vi "Parse Instructions.vi"(8 "error in (no error)":errorcluster, 11 "Instructions XML":string="<?xml version=\"1.0\" encoding=\"UTF-8\"?><ns2:instructions xmlns:ns2=\"http://jazz.net/xmlns/alm/qm/v0.1/\" xmlns:ns1=\"http://schema.ibm.com/vega/2008/\" xmlns:ns3=\"http://purl.org/dc/elements/1.1/\" xmlns:ns4=\"http://jazz.net/xmlns/prod/jazz/process/0.6/\" xmlns:ns5=\"http://jazz.net/xmlns/alm/v0.1/\" xmlns:ns6=\"http://www.w3.org/1999/02/22-rdf-syntax-ns#\" xmlns:ns7=\"http://purl.org/dc/terms/\" xmlns:ns8=\"http://jazz.net/xmlns/alm/qm/v0.1/tsl/v0.1/\" xmlns:ns9=\"http://jazz.net/xmlns/alm/qm/v0.1/testscript/v0.1/\" xmlns:ns10=\"http://jazz.net/xmlns/alm/qm/qmadapter/task/v0.1\" xmlns:ns11=\"http://jazz.net/xmlns/alm/qm/qmadapter/v0.1\" xmlns:ns12=\"http://jazz.net/xmlns/alm/qm/v0.1/executionworkitem/v0.1\" xmlns:ns13=\"http://jazz.net/xmlns/alm/qm/v0.1/executionresult/v0.1\" xmlns:ns14=\"http://jazz.net/xmlns/alm/qm/v0.1/catalog/v0.1\" xmlns:ns16=\"http://jazz.net/xmlns/alm/qm/styleinfo/v0.1/\" xmlns:ns17=\"http://www.w3.org/1999/XSL/Transform\"><ns11:workavailable>false</ns11:workavailable></ns2:instructions>") -> (0 "error out":errorcluster, 1 "Instructions":T1[](array[typedef]), 2 "Work available":bool)   [LabVIEW 2012]
uses:
  Instruction Info.ctl
  <vilib>/xml/Load XML String.vi
  <vilib>/xml/Close Reference(Node).vi
  <vilib>/xml/Close Reference(NdList).vi
  <vilib>/xml/NI_XML.lvlib
  <resource>/objmgr/DOMUserDefRef.rc
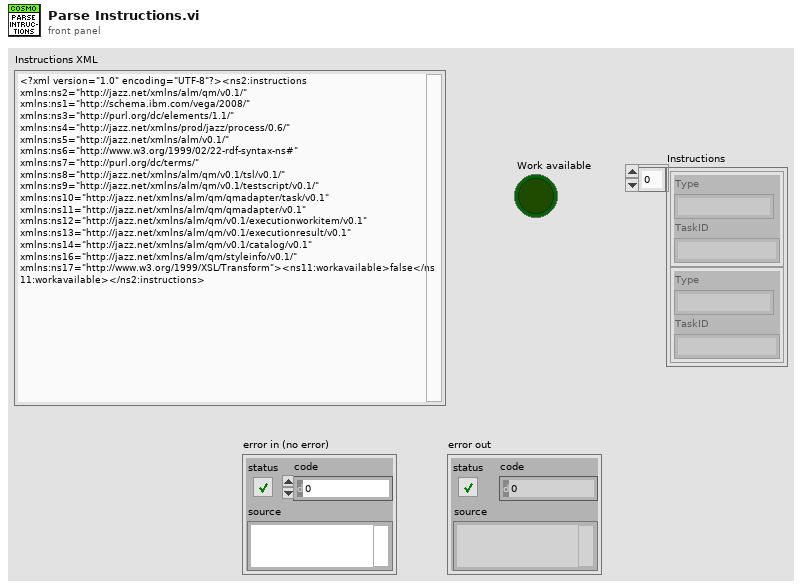
[diagram p1: front panel]
types:
  T1 = typedef "Instruction Info.ctl" = cluster{"Type":string, "TaskID":string}
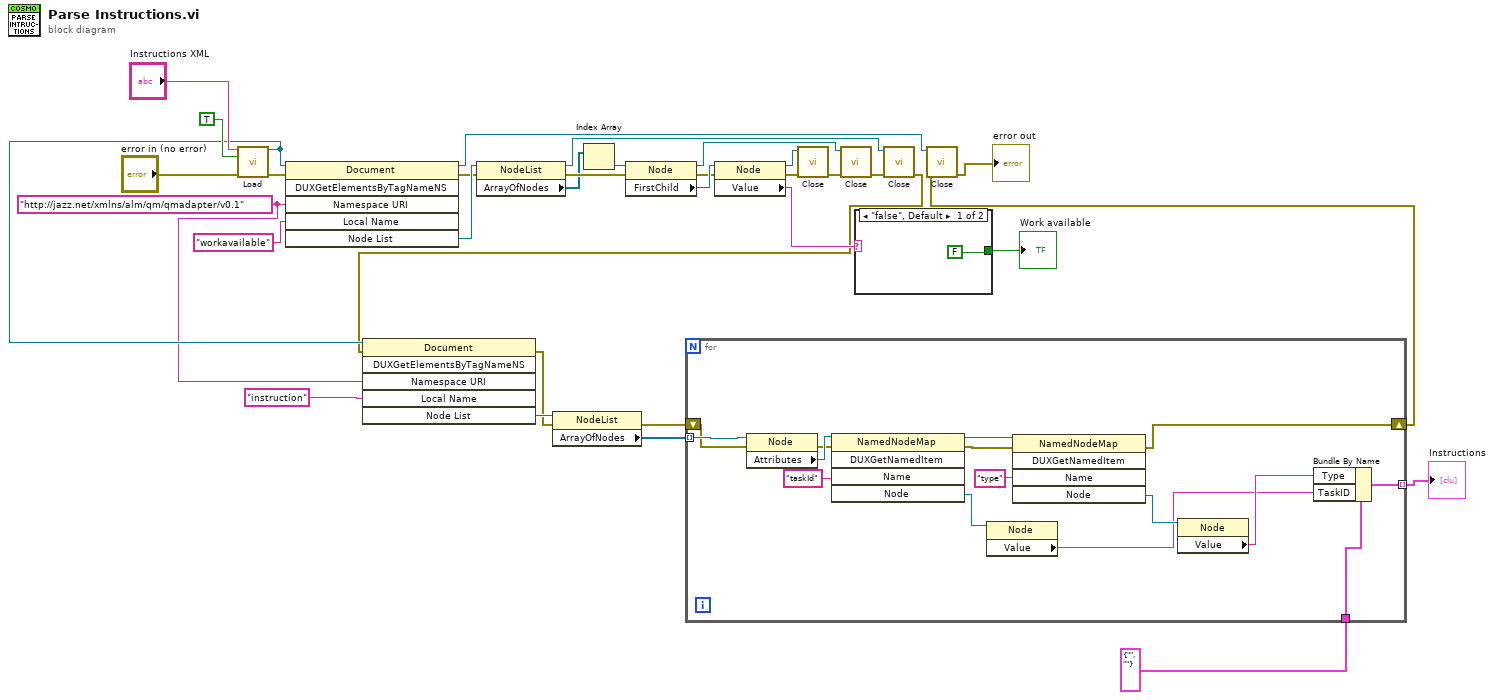
[diagram p0: block diagram]
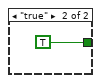
[diagram p2: hidden frame]
diagram:
  w11 = "http://jazz.net/xmlns/alm/qm/qmadapter/v0.1" ("Namespace URI")
  n1 = call-poly <vilib>:"Load.vi"("XML string"="Instructions XML", "process namespaces (False)"=TRUE, "error in (no error)"="error in (no error)") -> ("DOM document out"=w12:refnum<k20>, "error out"=w28:errorcluster)  [unwired: 10 in, 1 out]
  n2 = invoke class="Document" method="DUXGetElementsByTagNameNS"(reference=w12, error in=w28, "Namespace URI"=w11, "Local Name"="workavailable") -> (reference out=w21:refnum<k20>, error out=w29:errorcluster, "Node List"=w30:refnum<k20>)  [unwired: 2 in, 3 out]
  n3 = property class="NodeList"(reference=w30, error in=w29) -> (reference out=w27:refnum<k20>, error out=w24:errorcluster, "ArrayOfNodes"=w13:refnum<k20>[])
  n4 = Index Array(array=w13) -> (element=w25:refnum<k20>)  [unwired: 1 in]
  n5 = property class="Node"(reference=w25, error in=w24) -> (reference out=w22:refnum<k20>, error out=w19:errorcluster, "FirstChild"=w20:refnum<k20>)
  n6 = property class="Node"(reference=w20, error in=w19) -> (reference out=w18:refnum<k20>, error out=w17:errorcluster, "Value"=w15:string)
  n7 = call-poly <vilib>:"Close.vi"("error in (no error)"=w17, "node"=w18) -> ("error out"=w16:errorcluster)  [unwired: 7 in]
  n8 = call-poly <vilib>:"Close.vi"("error in (no error)"=w16, "node"=w22) -> ("error out"=w26:errorcluster)  [unwired: 7 in]
  n9 = case shown="\"false\", Default" w15 {
    tunnel: [FALSE TRUE] -> w14
    frame "false", Default {
    }
    frame "true" {
    }
  }
  "Work available" <- w14
  n10 = call-poly <vilib>:"Close.vi"("error in (no error)"=w26, "node list"=w27) -> ("error out"=w5:errorcluster)  [unwired: 7 in]
  n11 = invoke class="Document" method="DUXGetElementsByTagNameNS"(reference=w12, error in=w5, "Namespace URI"=w11, "Local Name"="instruction") -> (error out=w4:errorcluster, "Node List"=w9:refnum<k20>)  [unwired: 2 in, 4 out]
  n12 = property class="NodeList"(reference=w9, error in=w4) -> (error out=w3:errorcluster, "ArrayOfNodes"=w8:refnum<k20>[])  [unwired: 1 out]
  n13 = for {
    tunnel: w8 -> [w43] mode=indexing
    tunnel: T1 {"Type"="", "TaskID"=""} ("Intruction") -> [w42]
    tunnel: [w39] -> w6 mode=indexing
    shift-right: [w36] -> w2
    shift-left: w3 -> [w38]
    n14 = property class="Node"(reference=w43, error in=w38) -> (error out=w37:errorcluster, "Attributes"=w50:refnum<k20>)  [unwired: 1 out]
    n15 = invoke class="NamedNodeMap" method="DUXGetNamedItem"(reference=w50, error in=w37, "Name"="taskId") -> (reference out=w48:refnum<k20>, error out=w47:errorcluster, "Node"=w45:refnum<k20>)  [unwired: 2 in, 2 out]
    n16 = property class="Node"(reference=w45) -> ("Value"=w40:string)  [unwired: 1 in, 2 out]
    n17 = invoke class="NamedNodeMap" method="DUXGetNamedItem"(reference=w48, error in=w47, "Name"="type") -> (error out=w36:errorcluster, "Node"=w44:refnum<k20>)  [unwired: 2 in, 3 out]
    n18 = property class="Node"(reference=w44) -> ("Value"=w41:string)  [unwired: 1 in, 2 out]
    n19 = Bundle By Name(cluster=w42, "Type"=w41, "TaskID"=w40) -> (w39:T1)
  }
  "Instructions" <- w6
  n20 = call-poly <vilib>:"Close.vi"("error in (no error)"=w2, "node"=w21) -> ("error out"=→"error out":errorcluster)  [unwired: 7 in]
